vi "List Objects.vi"(4 "Region":T2, 7 "Max keys":u32, 8 "error in (no error)":errorcluster, 9 "Bucket":string, 10 "Delimiter":string, 11 "Prefix":string) -> (0 "error out":errorcluster, 1 "CommonPrefixes":T1[](array[typedef]), 3 "Contents":T3[](array[typedef]))   [LabVIEW 2015, in "LV Interface for Amazon S3.lvlib"]
doc: "This operation <B>returns some or all (default)</B> of the <B>objects</B> in a bucket. To use this operation, you <B>must have READ access</B> to the bucket."
uses:
  LV Interface for Amazon S3.lvlib
  Typedefs/AMZ_S3_API_ListBucketResult Content.ctl
  Typedefs/AMZ_S3_Storage Class.ctl
  Typedefs/AMZ_S3_API_Owner.ctl
  Typedefs/AMZ_S3_LocationConstraint.ctl
  Typedefs/AMZ_S3_API_ListBucketResult CommonPrefix.ctl
  Typedefs/AMZ_S3_API_GET Bucket Request Parameters.ctl
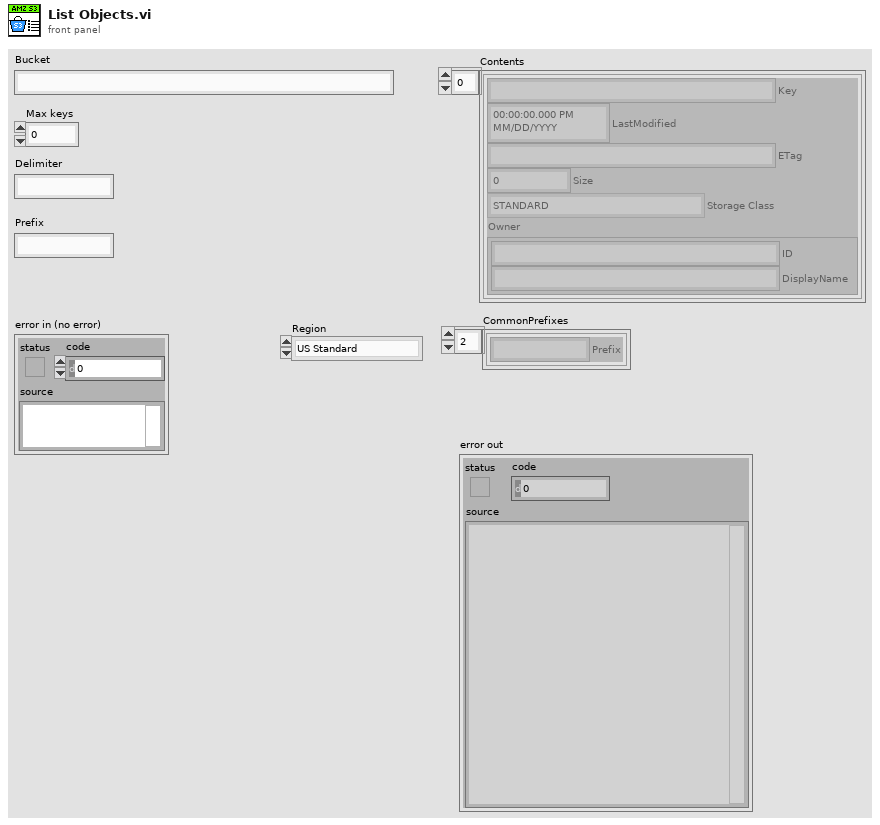
[diagram p1: front panel]
types:
  T1 = typedef "LV Interface for Amazon S3.lvlib/AMZ_S3_API_ListBucketResult CommonPrefix.ctl" = cluster{"Prefix":string}
  T2 = typedef "LV Interface for Amazon S3.lvlib/AMZ_S3_LocationConstraint.ctl" = enum16{"US Standard", "us-east-2", "us-west-1", "us-west-2", "ap-northeast-1", "ap-northeast-2", "ap-southeast-1", "ap-southeast-2", "ca-central-1", "eu-central-1", "eu-west-1", "eu-west-2", "sa-east-1"}
  T3 = typedef "LV Interface for Amazon S3.lvlib/AMZ_S3_API_ListBucketResult Content.ctl" = cluster{"Key":string, "LastModified":timestamp, "ETag":string, "Size":u64, "Storage Class":T4, "Owner":T5}
  T4 = typedef "LV Interface for Amazon S3.lvlib/AMZ_S3_Storage Class.ctl" = enum16{"STANDARD", "REDUCED_REDUNDANCY"}
  T5 = typedef "LV Interface for Amazon S3.lvlib/AMZ_S3_API_Owner.ctl" = cluster{"ID":string, "DisplayName":string}
  T6 = typedef "LV Interface for Amazon S3.lvlib/AMZ_S3_API_GET Bucket Request Parameters.ctl" = cluster{"delimiter":string, "marker":string, "max-keys":u16, "prefix":string}
  T7 = typedef "LV Interface for Amazon S3.lvlib/AMZ_S3_API_ListBucketResult.ctl" = cluster{"Name":string, "Prefix":string, "Marker":string, "MaxKeys":u16, "IsTruncated?":bool, "Contents":T3[], "CommonPrefixes":T1[]}
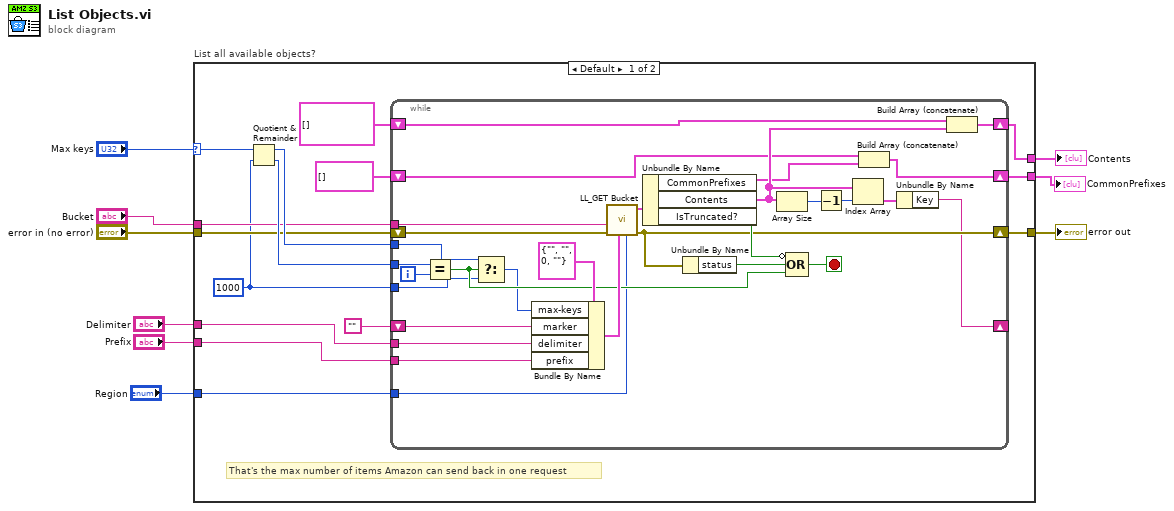
[diagram p0: block diagram]
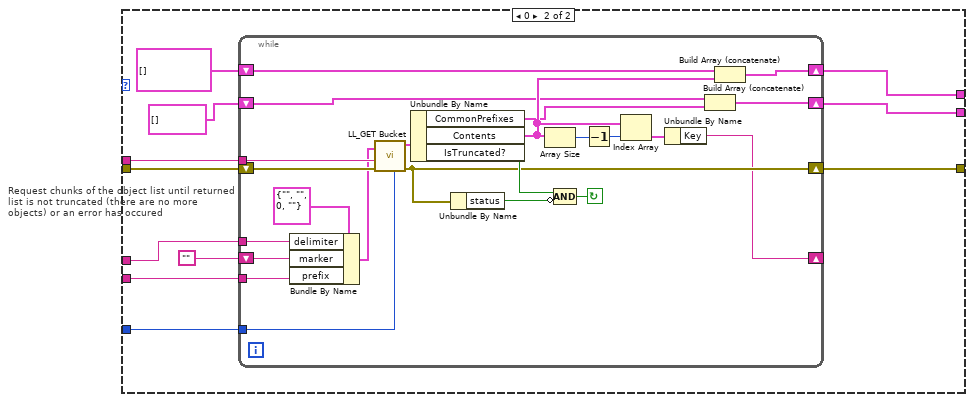
[diagram p2: hidden frame]
diagram:
  n1 = case "List all available objects?" shown="Default" "Max keys" {
    selector: "Max keys" -> [w24 _]
    tunnel: "error in (no error)" -> [w19 w64]
    tunnel: "Bucket" -> [w18 w63]
    tunnel: [w16 w61] -> w5
    tunnel: [w17 w59] -> w6
    tunnel: "Prefix" -> [w13 w58]
    tunnel: "Delimiter" -> [w14 w57]
    tunnel: "Region" -> [w12 w56]
    tunnel: [w11 w55] -> w1
    frame Default {
      w15 = u32 1000 ("y")
      # "That's the max number of items Amazon can send back in one request"
      n2 = Quotient & Remainder(x=w24, y=w15) -> (x-y*floor(x/y)=w20:u32, floor(x/y)=w21:u32)
      n3 = while {
        tunnel: w18 -> [w52]
        shift-right: [w48] -> w17
        shift-left: w19 -> [w53]
        shift-right: [w44] -> _
        shift-left: "" -> [w39]
        shift-right: [w42] -> w16
        shift-left: T3[] [] -> [w41]
        tunnel: w21 -> [w36]
        tunnel: w20 -> [w35]
        tunnel: w15 -> [w31]
        tunnel: w14 -> [w30]
        tunnel: w13 -> [w29]
        tunnel: w12 -> [w28]
        shift-right: [w26] -> w11
        shift-left: T1[] [] ("appended array") -> [w25]
        i -> [w37]
        stop <- w33 stop-if-true
        n4 = Equal?(x=w36, y=w37) -> (x = y?=w34:bool)
        n5 = Select(t=w35, s=w34, f=w31) -> (s? t:f=w32:u32)
        n6 = Bundle By Name(cluster=T6 {"delimiter"="", "marker"="", "max-keys"=0, "prefix"=""} ("GET Bucket Request Parameters"), "max-keys"=w32, "marker"=w39, "delimiter"=w30, "prefix"=w29) -> (w38:T6)
        n7 = call "LL_GET Bucket.vi"("Region"=w28, "GET Bucket Request Parameters"=w38, "error in (no error)"=w53, "Bucket"=w52) -> ("error out"=w48:errorcluster, "ListBucketResult"=w51:T7)  [unwired: 5 in, 1 out]
        n8 = Unbundle By Name(w51) -> ("CommonPrefixes"=w27:T1[], "Contents"=w43:T3[], "IsTruncated?"=w50:bool)
        n9 = Unbundle By Name(w48) -> ("status"=w49:bool)
        n10 = Array Size(array=w43) -> (size(s)=w47:i32)
        n11 = Compound Arithmetic op=OR(invert w50, w49, w34) -> (w33:bool)
        n12 = Decrement(x=w47) -> (x-1=w46:i32)
        n13 = Index Array(array=w43, index=w46) -> (element=w45:T3)
        n14 = Build Array (concatenate)(w25, w27) -> (w26:T1[])
        n15 = Unbundle By Name(w45) -> ("Key"=w44:string)
        n16 = Build Array (concatenate)(w41, w43) -> (w42:T3[])
      }
    }
    frame 0 {
      n17 = while "Request chunks of the object list until returned list is not truncated (there are no more objects) or an error has occured" {
        tunnel: w63 -> [w86]
        shift-right: [w81] -> w59
        shift-left: w64 -> [w87]
        shift-right: [w77] -> _
        shift-left: "" -> [w72]
        shift-right: [w75] -> w61
        shift-left: T3[] [] -> [w74]
        tunnel: w58 -> [w70]
        tunnel: w57 -> [w69]
        tunnel: w56 -> [w68]
        shift-right: [w67] -> w55
        shift-left: T1[] [] -> [w65]
        stop <- w82 continue-if-true
        n18 = Bundle By Name(cluster=T6 {"delimiter"="", "marker"="", "max-keys"=0, "prefix"=""} ("GET Bucket Request Parameters"), "delimiter"=w69, "marker"=w72, "prefix"=w70) -> (w71:T6)
        n19 = call "LL_GET Bucket.vi"("Region"=w68, "GET Bucket Request Parameters"=w71, "error in (no error)"=w87, "Bucket"=w86) -> ("error out"=w81:errorcluster, "ListBucketResult"=w85:T7)  [unwired: 5 in, 1 out]
        n20 = Unbundle By Name(w85) -> ("CommonPrefixes"=w66:T1[], "Contents"=w76:T3[], "IsTruncated?"=w84:bool)
        n21 = Unbundle By Name(w81) -> ("status"=w83:bool)
        n22 = Array Size(array=w76) -> (size(s)=w80:i32)
        n23 = Compound Arithmetic op=AND(w84, invert w83) -> (w82:bool)
        n24 = Decrement(x=w80) -> (x-1=w79:i32)
        n25 = Index Array(array=w76, index=w79) -> (element=w78:T3)
        n26 = Unbundle By Name(w78) -> ("Key"=w77:string)
        n27 = Build Array (concatenate)(w65, w66) -> (w67:T1[])
        n28 = Build Array (concatenate)(w74, w76) -> (w75:T3[])
      }
    }
  }
  "error out" <- w6
  "Contents" <- w5
  "CommonPrefixes" <- w1
